vi "MongoDB.GetCollection.vi"(8 "error in (no error)":errorcluster, 10 "collectionName":string, 11 "MongoDB.Database in":refnum<class "MongoDB.Database.lvclass">) -> (0 "error out":errorcluster, 2 "MongoDB.Collection out":refnum<class "MongoDB.Collection.lvclass">, 3 "MongoDB.Database out":refnum<class "MongoDB.Database.lvclass">)   [LabVIEW 2014, in "MongoDB.Database.lvclass"]
uses:
  MongoDB.Database.lvclass
  MongoDB.Collection.lvclass
  MongoDB.Database.lvclass/MongoDB.Database.ctl
  C:/Users/Richard/Documents/GitHub/mongo-labview-driver/CSharp/bin/MongoDB.Driver.Legacy.dll
  CSharp/bin/MongoDB.Driver.Legacy.dll
  MongoDB.Collection.lvclass/MongoDB.Collection.ctl
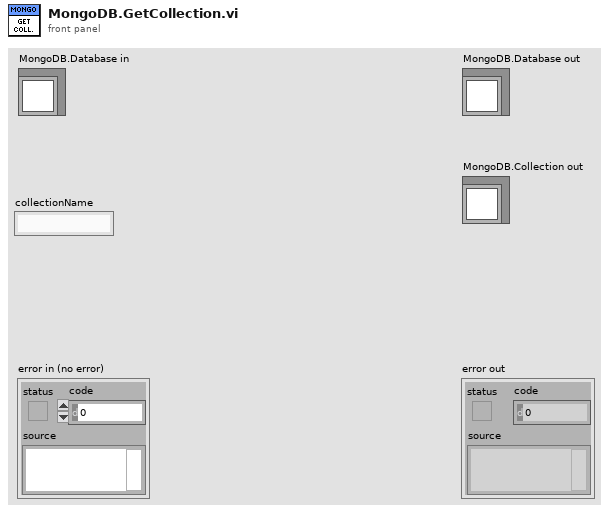
[diagram p1: front panel]
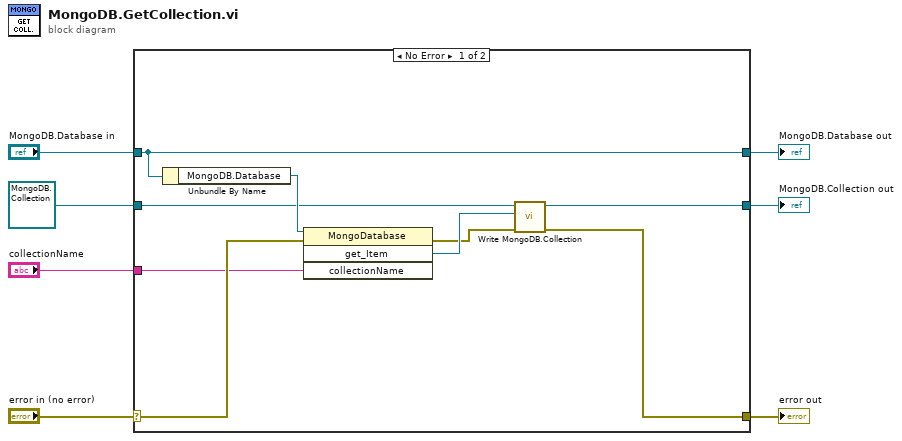
[diagram p0: block diagram]
diagram:
  n1 = case shown="No Error" "error in (no error)" {
    selector: "error in (no error)" -> [w15 w19]
    tunnel: [w12 w19] -> w6
    tunnel: [w9 w18] -> w4
    tunnel: "MongoDB.Database in" -> [w9 w18]
    tunnel: [w11 w17] -> w3
    tunnel: refnum<class "MongoDB.Collection.lvclass"> refnum ("MongoDB.Collection in") -> [w10 w17]
    tunnel: "collectionName" -> [w8 _]
    frame No Error {
      n2 = Unbundle By Name(w9) -> ("MongoDB.Database"=w16:refnum<k24>)
      n3 = invoke class="MongoDatabase" method="get_Item"(reference=w16, error in=w15, "collectionName"=w8) -> (error out=w13:errorcluster, "get_Item"=w14:refnum<k24>)  [unwired: 1 in, 2 out]
      n4 = call "Write MongoDB.Collection.vi"("error in (no error)"=w13, "MongoDB.Collection"=w14, "MongoDB.Collection in"=w10) -> ("error out"=w12:errorcluster, "MongoDB.Collection out"=w11:refnum<class "MongoDB.Collection.lvclass">)  [unwired: 7 in]
    }
    frame Error {
    }
  }
  "error out" <- w6
  "MongoDB.Database out" <- w4
  "MongoDB.Collection out" <- w3
